vi "copy Data to Array 2D.vi"(4 "error in (no error)":errorcluster, 7 "Data in":refnum<class "Data.lvclass">) -> (0 "error out":errorcluster, 2 "Data Content":sgl[][](array[numeric]), 3 "Data out":refnum<class "Data.lvclass">)   [LabVIEW 2018]
uses:
  SpectralRadar/LabVIEW/2012/user.lib/SpectralRadar.llb/Data.lvclass
  SpectralRadar/LabVIEW/2012/user.lib/SpectralRadar.llb/Data Property Int Selection.ctl
  SpectralRadar/LabVIEW/2012/user.lib/SpectralRadar.llb/get Data Property Int.vi
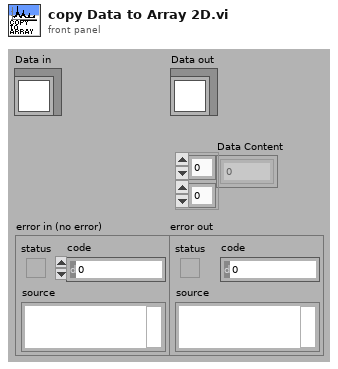
[diagram p1: front panel]
types:
  T1 = typedef "Data.lvclass/Data Property Int Selection.ctl" = enum16{"Dimensions", "Size 1", "Size 2", "Size 3", "Number of Data Points", "Data Size in Bytes", "Bytes per Pixel"}
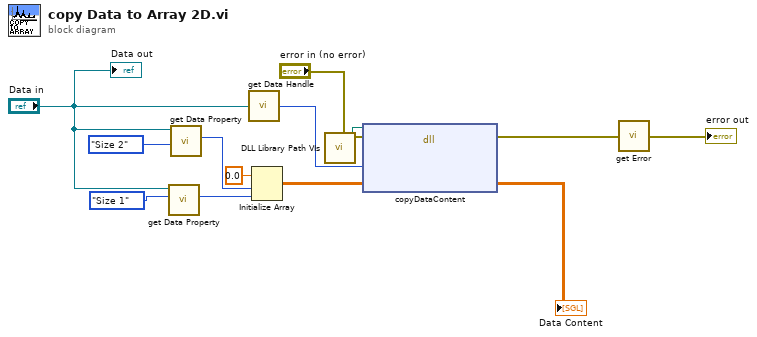
[diagram p0: block diagram]
diagram:
  n1 = call-poly "get Data Property.vi"("Data Property Selection"=Data_Property_Int_Selection."Size 1", "Data"="Data in") -> ("Property Value"=w6:i32)  [unwired: 3 in, 2 out]
  n2 = call-poly "get Data Property.vi"("Data Property Selection"=Data_Property_Int_Selection."Size 2", "Data"="Data in") -> ("Property Value"=w5:i32)  [unwired: 3 in, 2 out]
  n3 = call "get Data Handle.vi"("Data"="Data in") -> ("Handle"=w12:u64)
  n4 = Initialize Array(sgl 0.0 ("element"), w5, w6) -> (w11:sgl[][])
  n5 = call "DLL Library Path VIs.vi"() -> ("SpectralRadarDLL"=w1:path)  [unwired: 8 in, 3 out]
  n6 = dll-call lib="C:/Project/SerialSectOCT - FFT GPU/SerialSectOCT/Labview Software/DLL/SpectralRadar.dll" fn="copyDataContent"(path in=w1, error in="error in (no error)", "Data Handle"=w12, "Data Content"=w11) -> (error out=w3:errorcluster, "Data Content"=→"Data Content":sgl[][])  [unwired: 3 in, 1 out]
  n7 = call "get Error.vi"("error in (no error)"=w3) -> ("error out"=→"error out":errorcluster)
  "Data out" <- "Data in"
